vi "String Constant - Inside JKI SM.vi"() -> ()   [LabVIEW 2020]
panel:
  in  "OK":bool
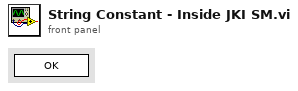
[diagram p1: front panel]
types:
  T1 = enum32{"invalid app kind", "Development System", "Run Time System", "Student Edition", "Embedded LabVIEW", "Evaluation", "Custom"}
  T2 = enum32{"Invalid", "Standard", "Closed", "Hidden", "Minimized", "Maximized"}
  T3 = cluster{"Core":cluster{"Current VI Reference":refnum<vi>, "Close Panel on Exit?":bool}, "Your Boolean data":bool}
  T4 = cluster{"Current VI Reference":refnum<vi>, "Close Panel on Exit?":bool}
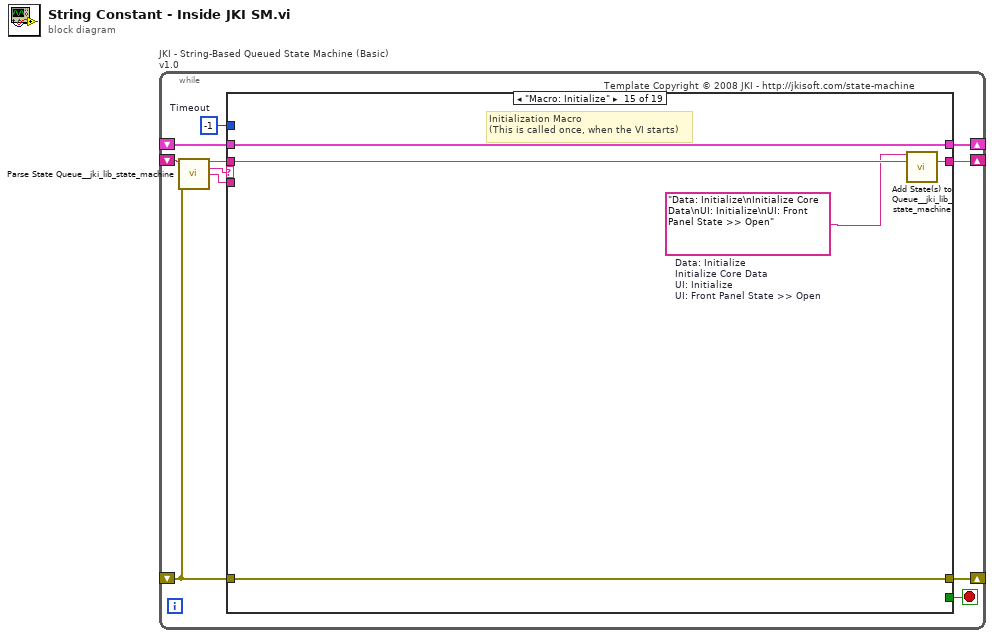
[diagram p0: block diagram]
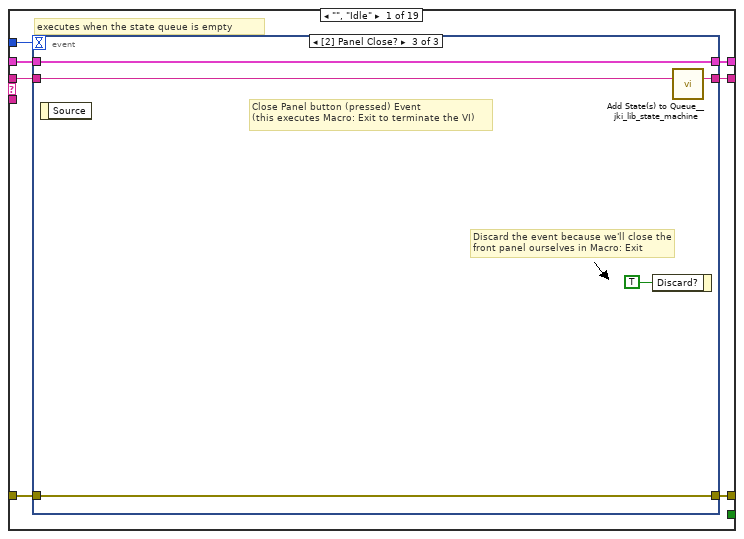
[diagram p2: hidden frame]
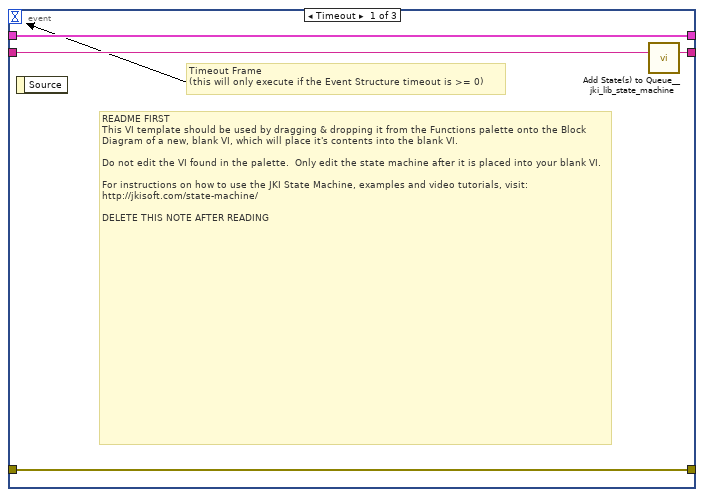
[diagram p3: hidden frame]
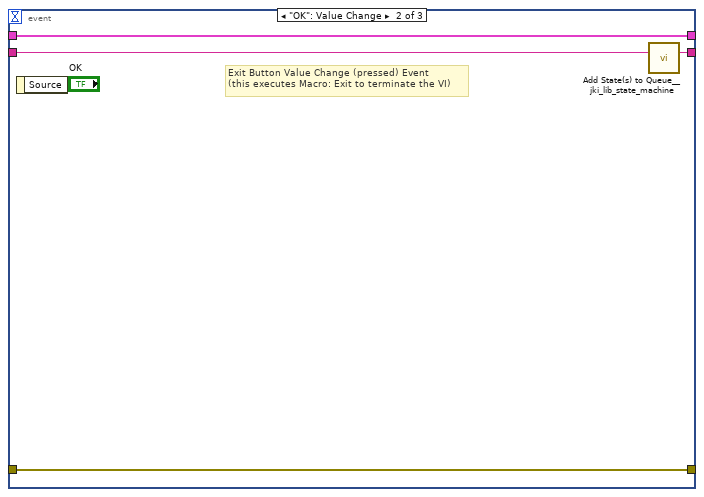
[diagram p4: hidden frame]
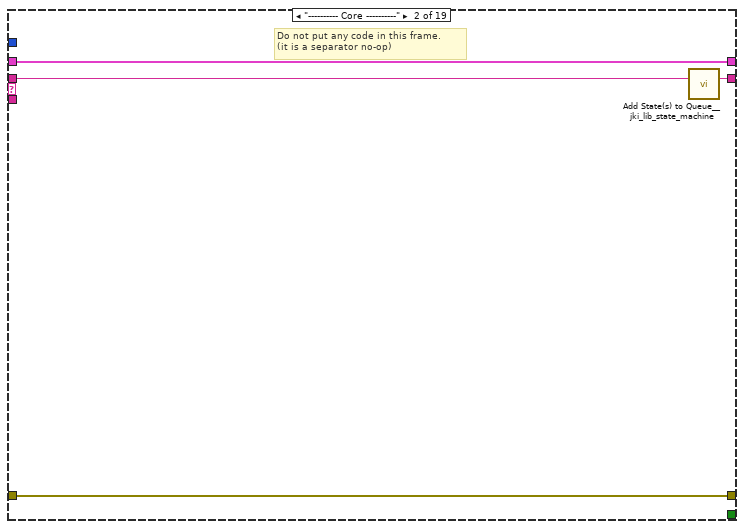
[diagram p5: hidden frame]
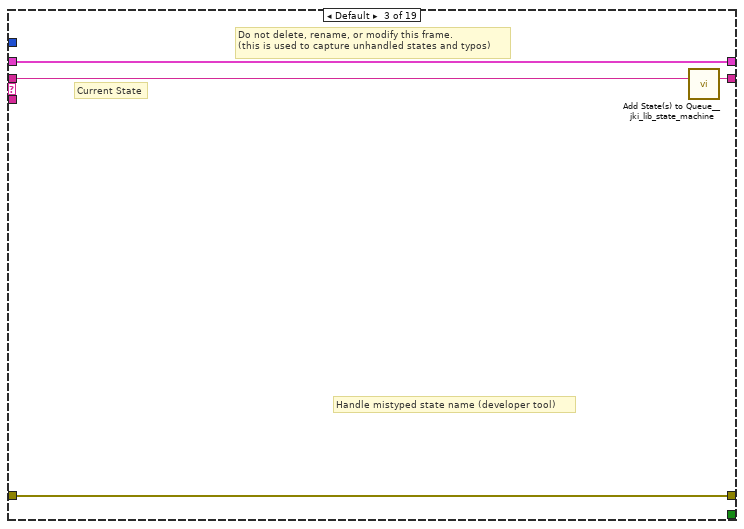
[diagram p6: hidden frame]
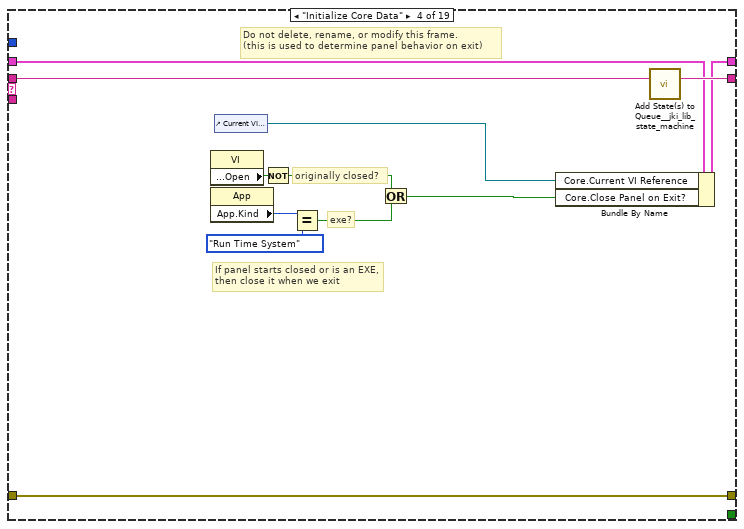
[diagram p7: hidden frame]
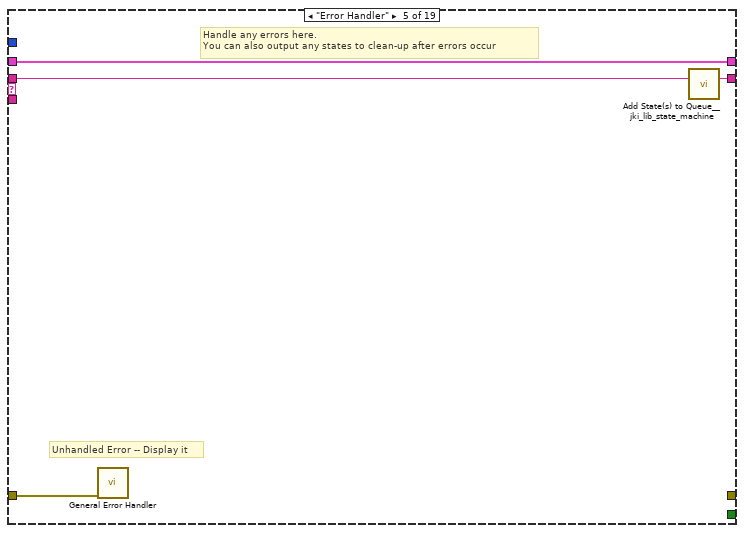
[diagram p8: hidden frame]
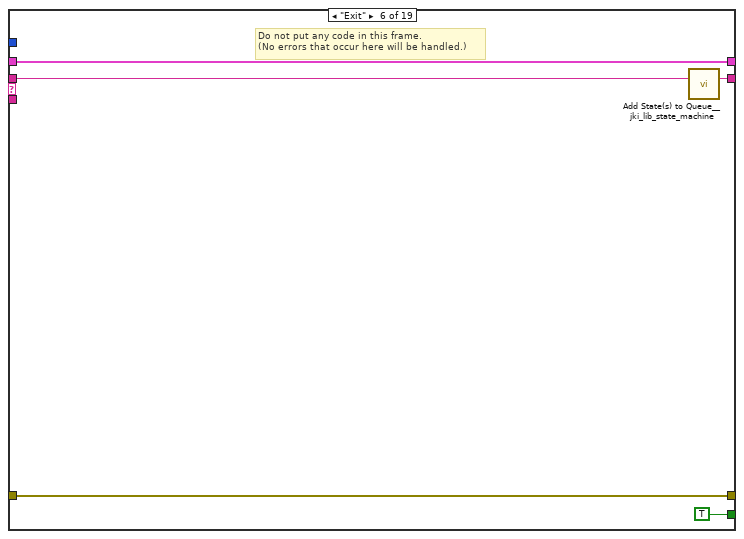
[diagram p9: hidden frame]
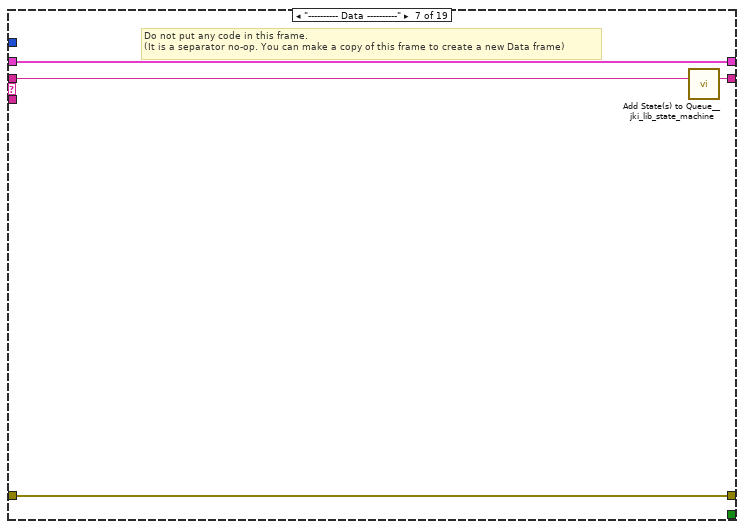
[diagram p10: hidden frame]
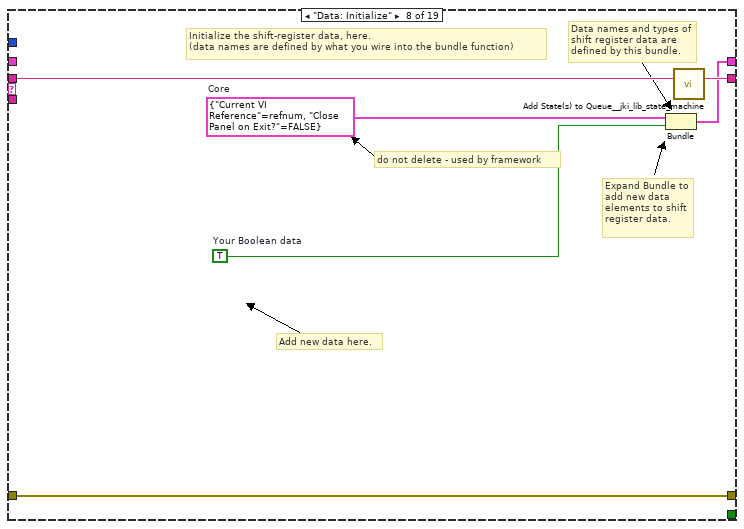
[diagram p11: hidden frame]
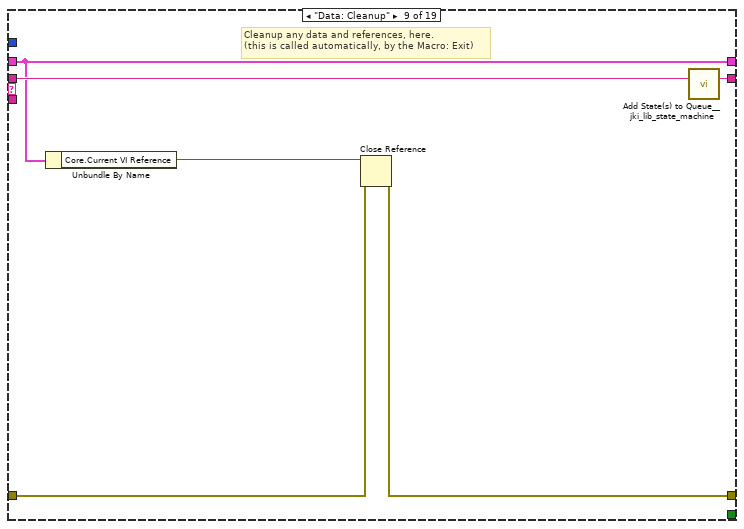
[diagram p12: hidden frame]
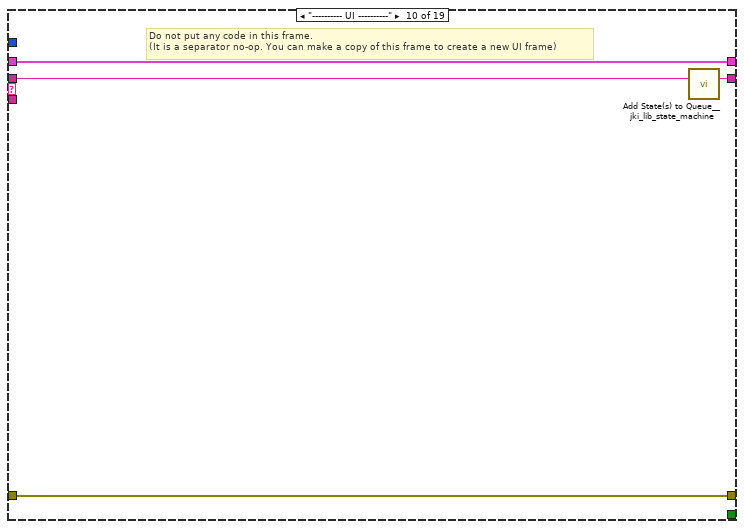
[diagram p13: hidden frame]
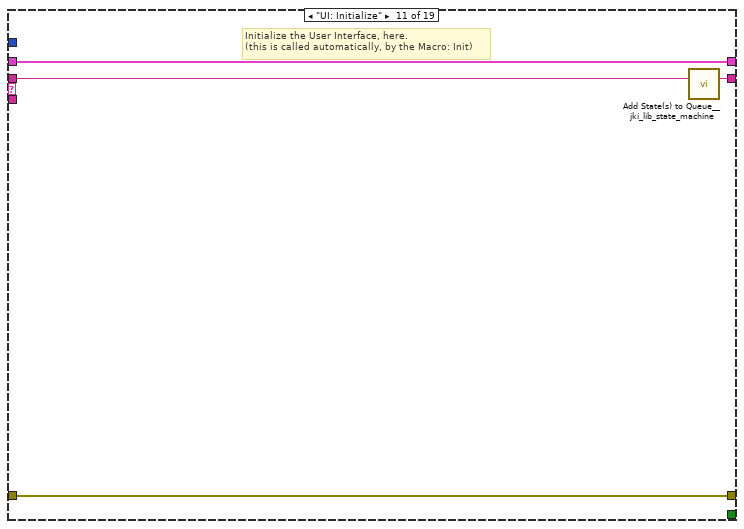
[diagram p14: hidden frame]
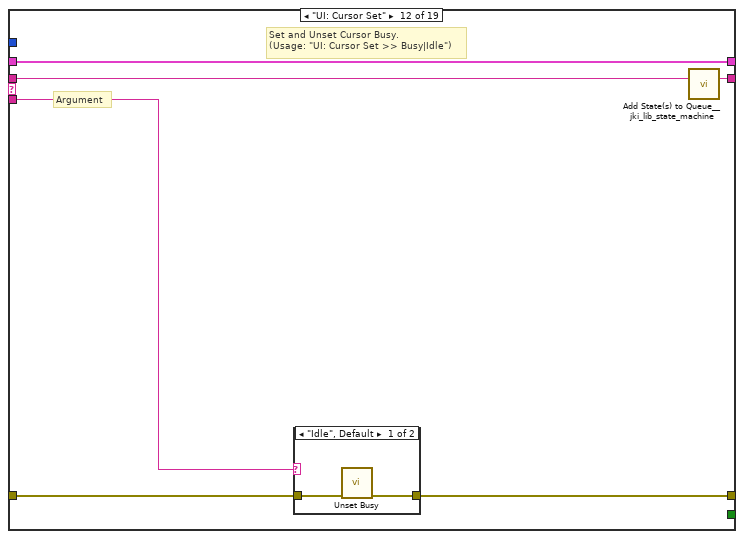
[diagram p15: hidden frame]
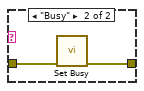
[diagram p16: hidden frame]
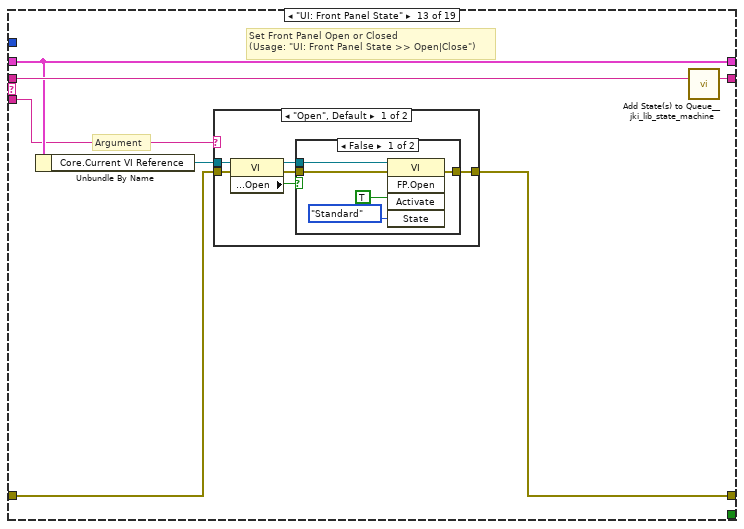
[diagram p17: hidden frame]
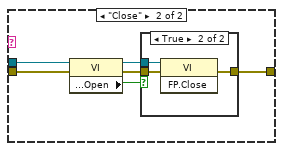
[diagram p19: hidden frame]
diagram:
  n1 = while "JKI - String-Based Queued State Machine (Basic) v1.0" {
    shift-right: [w4] -> _
    shift-left: _ -> [w3]
    shift-right: [w7] -> _
    shift-left: _ -> [w1]
    shift-right: [w6] -> _
    shift-left: _ -> [w8]
    stop <- w5 stop-if-true
    w2 = -1  # Timeout
    # "Template Copyright © 2008 JKI - http://jkisoft.com/state-machine"
    n2 = call <vilib>:"Parse State Queue__jki_lib_state_machine.vi"("State Queue"=w8, "Error In (no error)"=w1) -> ("Remaining States"=w10:string, "Current State"=w11:string, "Arguments"=w9:string)  [unwired: 11 in]
    n3 = case shown="\"Macro: Initialize\"" w11 {
      tunnel: w10 -> [w18 w35 w38 w51 w55 w60 w64 w70 w76 w80 w84 w90 w101 w127 w132 w136 w140 w144 w148]
      tunnel: w9 -> [_ _ _ _ _ _ _ _ _ _ _ w85 w95 _ _ _ _ _ _]
      tunnel: w3 -> [w16 w32 w36 w42 w53 w58 w61 _ w71 w77 w82 w88 w97 w124 w129 w133 w137 w141 w145]
      tunnel: [w15 w33 w39 w48 _ w57 w62 w67 w72 w78 w81 w86 w98 w125 w130 w134 w138 w142 w146] -> w7
      tunnel: w1 -> [w14 w33 w39 w48 w52 w57 w62 w67 w73 w78 w81 w87 w99 w125 w130 w134 w138 w142 w146]
      tunnel: [w17 w34 w37 w50 w54 w59 w63 w69 w75 w79 w83 w89 w100 w126 w131 w135 w139 w143 w147] -> w6
      tunnel: [_ _ _ _ _ TRUE _ _ _ _ _ _ _ _ _ _ _ _ _] -> w5
      tunnel: [w13 w32 w36 w49 w53 w58 w61 w68 w71 w77 w82 w88 w97 w124 w129 w133 w137 w141 w145] -> w4
      tunnel: w2 -> [w12 _ _ _ _ _ _ _ _ _ _ _ _ _ _ _ _ _ _]
      frame "", "Idle" {
        # "executes when the state queue is empty"
        n4 = event shown="[2] Panel Close?" {
          selector: _ -> [_ _ _]
          dyn-events: _ -> [_ _ _]
          timeout: w12 -> [_ _ _]
          tunnel: w18 -> [w22 w26 w31]
          tunnel: [w21 w25 w30] -> w17
          tunnel: w16 -> [w19 w23 w28]
          tunnel: [w20 w24 w29] -> w15
          tunnel: w14 -> [w20 w24 w29]
          tunnel: [w19 w23 w28] -> w13
          event Timeout {
            # "README FIRST\nThis VI template should be used by dragging & dropping it from the Functions palette onto the Block Diagram of a new, blank VI, which will place it's contents into the blank VI.\n\nDo not edit the VI found in the palette.  Only edit the state machine after it is placed into your blank VI.\n\nFor instructions on how to use the JKI State Machine, examples and video tutorials, visit:\nhttp://jkisoft.com/state-machine/\n\nDELETE THIS NOTE AFTER READING"
            # "Timeout Frame\n(this will only execute if the Event Structure timeout is >= 0)"
            n5 = event-data() -> ()  [unwired: 1 in, 1 out]
            n6 = call <vilib>:"Add State(s) to Queue__jki_lib_state_machine.vi"("State(s) in (\"\")"=w22) -> ("States Out"=w21:string)  [unwired: 14 in]
          }
          event "OK": Value Change {
            # "Exit Button Value Change (pressed) Event\n(this executes Macro: Exit to terminate the VI)"
            n7 = event-data() -> ()  [unwired: 1 in, 1 out]
            n8 = call <vilib>:"Add State(s) to Queue__jki_lib_state_machine.vi"("State(s) in (\"\")"=w26) -> ("States Out"=w25:string)  [unwired: 14 in]
          }
          event Panel Close? {
            # "Discard the event because we'll close the front panel ourselves in Macro: Exit"
            # "Close Panel button (pressed) Event\n(this executes Macro: Exit to terminate the VI)"
            n9 = event-data() -> ()  [unwired: 1 in, 1 out]
            n10 = event-data("Discard?"=TRUE) -> ()  [unwired: 1 in, 1 out]
            n11 = call <vilib>:"Add State(s) to Queue__jki_lib_state_machine.vi"("State(s) in (\"\")"=w31) -> ("States Out"=w30:string)  [unwired: 14 in]
          }
        }
      }
      frame "---------- Core ----------" {
        # "Do not put any code in this frame.\n(it is a separator no-op)"
        n12 = call <vilib>:"Add State(s) to Queue__jki_lib_state_machine.vi"("State(s) in (\"\")"=w35) -> ("States Out"=w34:string)  [unwired: 14 in]
      }
      frame Default {
        # "Current State"
        # "Do not delete, rename, or modify this frame.\n(this is used to capture unhandled states and typos)"
        # "Handle mistyped state name (developer tool)"
        n13 = call <vilib>:"Add State(s) to Queue__jki_lib_state_machine.vi"("State(s) in (\"\")"=w38) -> ("States Out"=w37:string)  [unwired: 14 in]
      }
      frame "Initialize Core Data" {
        # "Do not delete, rename, or modify this frame.\n(this is used to determine panel behavior on exit)"
        # "originally closed?"
        # "exe?"
        # "If panel starts closed or is an EXE, then close it when we exit"
        n14 = property class="VI"() -> ("Front Panel.Open"=w47:bool)  [unwired: 2 in, 2 out]
        n15 = property class="App"() -> ("App.Kind"=w46:T1)  [unwired: 2 in, 2 out]
        n16 = control-ref of="Current VI Reference"() -> (w40:refnum<vi>)
        n17 = Not(x=w47) -> (.not. x?=w44:bool)
        n18 = Equal?(x=w46, y=T1."Run Time System" ("Application:Kind")) -> (x = y?=w43:bool)
        n19 = Or(x=w44, y=w43) -> (x .or. y?=w41:bool)
        n20 = Bundle By Name(cluster=w42, "Core.Current VI Reference"=w40, "Core.Close Panel on Exit?"=w41) -> (w49:T3)
        n21 = call <vilib>:"Add State(s) to Queue__jki_lib_state_machine.vi"("State(s) in (\"\")"=w51) -> ("States Out"=w50:string)  [unwired: 14 in]
      }
      frame "Error Handler" {
        # "Unhandled Error -- Display it"
        # "Handle any errors here.\nYou can also output any states to clean-up after errors occur"
        n22 = call <vilib>:"General Error Handler.vi"("error in (no error)"=w52) -> ()  [unwired: 10 in, 5 out]
        n23 = call <vilib>:"Add State(s) to Queue__jki_lib_state_machine.vi"("State(s) in (\"\")"=w55) -> ("States Out"=w54:string)  [unwired: 14 in]
      }
      frame "Exit" {
        # "Do not put any code in this frame.\n(No errors that occur here will be handled.)"
        n24 = call <vilib>:"Add State(s) to Queue__jki_lib_state_machine.vi"("State(s) in (\"\")"=w60) -> ("States Out"=w59:string)  [unwired: 14 in]
      }
      frame "---------- Data ----------" {
        # "Do not put any code in this frame.\n(It is a separator no-op. You can make a copy of this frame to create a new Data frame)"
        n25 = call <vilib>:"Add State(s) to Queue__jki_lib_state_machine.vi"("State(s) in (\"\")"=w64) -> ("States Out"=w63:string)  [unwired: 14 in]
      }
      frame "Data: Initialize" {
        w65 = T4 {"Current VI Reference"=refnum, "Close Panel on Exit?"=FALSE}  # Core
        w66 = TRUE  # Your Boolean data
        # "do not delete - used by framework"
        # "Expand Bundle to add new data elements to shift register data."
        # "Add new data here."
        # "Data names and types of shift register data are defined by this bundle."
        # "Initialize the shift-register data, here.\n(data names are defined by what you wire into the bundle function)"
        n26 = Bundle("Core"=w65, "Your Boolean data"=w66) -> (w68:T3)  [unwired: 1 in]
        n27 = call <vilib>:"Add State(s) to Queue__jki_lib_state_machine.vi"("State(s) in (\"\")"=w70) -> ("States Out"=w69:string)  [unwired: 14 in]
      }
      frame "Data: Cleanup" {
        # "Cleanup any data and references, here.\n(this is called automatically, by the Macro: Exit)"
        n28 = Unbundle By Name(w71) -> ("Core.Current VI Reference"=w74:refnum<vi>)
        n29 = Close Reference(reference=w74, error in (no error)=w73) -> (error out=w72:errorcluster)
        n30 = call <vilib>:"Add State(s) to Queue__jki_lib_state_machine.vi"("State(s) in (\"\")"=w76) -> ("States Out"=w75:string)  [unwired: 14 in]
      }
      frame "---------- UI ----------" {
        # "Do not put any code in this frame.\n(It is a separator no-op. You can make a copy of this frame to create a new UI frame)"
        n31 = call <vilib>:"Add State(s) to Queue__jki_lib_state_machine.vi"("State(s) in (\"\")"=w80) -> ("States Out"=w79:string)  [unwired: 14 in]
      }
      frame "UI: Initialize" {
        # "Initialize the User Interface, here.\n(this is called automatically, by the Macro: Init)"
        n32 = call <vilib>:"Add State(s) to Queue__jki_lib_state_machine.vi"("State(s) in (\"\")"=w84) -> ("States Out"=w83:string)  [unwired: 14 in]
      }
      frame "UI: Cursor Set" {
        # "Argument"
        # "Set and Unset Cursor Busy.\n(Usage: \"UI: Cursor Set >> Busy|Idle\")"
        n33 = case shown="\"Idle\", Default" w85 {
          tunnel: w87 -> [w92 w94]
          tunnel: [w91 w93] -> w86
          frame "Idle", Default {
            n34 = call <vilib>:"Unset Busy.vi"("error in (no error)"=w92) -> ("error out"=w91:errorcluster)  [unwired: 10 in]
          }
          frame "Busy" {
            n35 = call <vilib>:"Set Busy.vi"("error in (no error)"=w94) -> ("error out"=w93:errorcluster)  [unwired: 9 in, 1 out]
          }
        }
        n36 = call <vilib>:"Add State(s) to Queue__jki_lib_state_machine.vi"("State(s) in (\"\")"=w90) -> ("States Out"=w89:string)  [unwired: 14 in]
      }
      frame "UI: Front Panel State" {
        # "Argument"
        # "Set Front Panel Open or Closed\n(Usage: \"UI: Front Panel State >> Open|Close\")"
        n37 = Unbundle By Name(w97) -> ("Core.Current VI Reference"=w96:refnum<vi>)
        n38 = case shown="\"Open\", Default" w95 {
          tunnel: w99 -> [w105 w118]
          tunnel: [w107 w119] -> w98
          tunnel: w96 -> [w106 w116]
          frame "Open", Default {
            n39 = property class="VI"(reference=w106, error in=w105) -> (reference out=w103:refnum<vi>, error out=w104:errorcluster, "Front Panel.Open"=w102:bool)
            n40 = case shown="False" w102 {
              tunnel: [w110 w113] -> w107
              tunnel: w104 -> [w109 w113]
              tunnel: w103 -> [w108 _]
              frame False {
                n41 = invoke class="VI" method="FP.Open"(reference=w108, error in=w109, "Activate"=TRUE, "State"=T2."Standard") -> (error out=w110:errorcluster)  [unwired: 1 in, 4 out]
              }
              frame True {
              }
            }
          }
          frame "Close" {
            n42 = property class="VI"(reference=w116, error in=w118) -> (reference out=w115:refnum<vi>, error out=w117:errorcluster, "Front Panel.Open"=w114:bool)
            n43 = case shown="True" w114 {
              tunnel: [w120 w123] -> w119
              tunnel: w117 -> [w120 w122]
              tunnel: w115 -> [_ w121]
              frame False {
              }
              frame True {
                n44 = invoke class="VI" method="FP.Close"(reference=w121, error in=w122) -> (error out=w123:errorcluster)  [unwired: 1 in, 2 out]
              }
            }
          }
        }
        n45 = call <vilib>:"Add State(s) to Queue__jki_lib_state_machine.vi"("State(s) in (\"\")"=w101) -> ("States Out"=w100:string)  [unwired: 14 in]
      }
      frame "---------- Macro ----------" {
        # "Do not put any code in this frame.\n(It is a separator no-op. You can make a copy of this frame to create a new Macro frame)"
        n46 = call <vilib>:"Add State(s) to Queue__jki_lib_state_machine.vi"("State(s) in (\"\")"=w127) -> ("States Out"=w126:string)  [unwired: 14 in]
      }
      frame "Macro: Initialize" {
        w128 = "Data: Initialize\nInitialize Core Data\nUI: Initialize\nUI: Front Panel State >> Open"  # Data: Initialize Initialize Core Data UI: Initialize UI: Front Panel State >> Open
        # "Initialization Macro\n(This is called once, when the VI starts)"
        n47 = call <vilib>:"Add State(s) to Queue__jki_lib_state_machine.vi"("State(s) in Front (\"\")"=w128, "State(s) in (\"\")"=w132) -> ("States Out"=w131:string)  [unwired: 13 in]
      }
      frame "Macro: Exit" {
        # "Exit Macro\n(This is called once, when the VI exits)"
        n48 = Unbundle By Name(w133) -> ()  [unwired: 1 out]
        n49 = call <vilib>:"Add State(s) to Queue__jki_lib_state_machine.vi"("State(s) in (\"\")"=w136) -> ("States Out"=w135:string)  [unwired: 14 in]
      }
      frame "---------- New Category ----------" {
        # "Template Separator\n(You can make a copy of, or modify, this frame)"
        n50 = call <vilib>:"Add State(s) to Queue__jki_lib_state_machine.vi"("State(s) in (\"\")"=w140) -> ("States Out"=w139:string)  [unwired: 14 in]
      }
      frame "New Category: 1" {
        # "Your code here.\n(You can make a copy of, or modify, this frame)"
        n51 = call <vilib>:"Add State(s) to Queue__jki_lib_state_machine.vi"("State(s) in (\"\")"=w144) -> ("States Out"=w143:string)  [unwired: 14 in]
      }
      frame "New Category: 2" {
        # "Your code here.\n(You can make a copy of, or modify, this frame)"
        n52 = call <vilib>:"Add State(s) to Queue__jki_lib_state_machine.vi"("State(s) in (\"\")"=w148) -> ("States Out"=w147:string)  [unwired: 14 in]
      }
    }
  }
